vi "KCSQ_Receive(SubVI).vi"(8 "error in (no error)":errorcluster) -> (0 "error out":errorcluster, 2 "Data":variant, 3 "Command":T1=enum."WaitOnReport")   [LabVIEW 2018, in "MainFrameLib.lvlib"]
uses:
  MainFrameLib.lvlib
  TypeDefs/Command_Enum.ctl
  TypeDefs/QNamesEnum.ctl
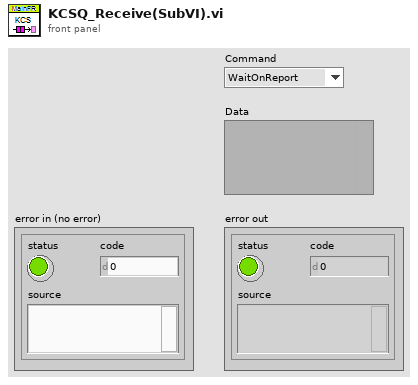
[diagram p1: front panel]
types:
  T1 = typedef "MainFrameLib.lvlib/Command_Enum.ctl" = enum16{"CheckSRLinks", "UpdateKCSColorCode", "StartLinkageCheck", "GetSRNotes", "DisplayAEStats", "InWork&Neglected", "RemapAENames", "ClearFolder", "UpdateReportsList", "ExcelReports", "TeamStats", "LoadReport", "WaitOnReport", "RequestReport", "Error", "Idle", "InitializeData", "ScreenPop", "Initialize", "UpdateCiscoAgentsView", "CancelRequests", "ClipboardCopy", "SaveNeglectedToFile", "Shutdown"}
  T2 = typedef "MainFrameLib.lvlib/QNamesEnum.ctl" = enum16{"UIQ", "ProcessQ", "CiscoQ", "KCSQ"}
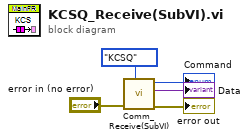
[diagram p0: block diagram]
diagram:
  n1 = call "Comm_Receive(SubVI).vi"("QueueSelector"=QNamesEnum."KCSQ" ("QueuSelector"), "Error In"="error in (no error)") -> ("error out"=→"error out":errorcluster, "Data"=→"Data":variant, "Command"=→"Command":T1)  [unwired: 7 in]
